vi "Write RS-xxx To GPIB ConvBox Data Structure.vi"(8 "error in (no error)":errorcluster, 10 "RS-xxx To GPIB ConvBox Data Structure":T1, 11 "Listener in":refnum<class "Listener.lvclass">) -> (0 "error out":errorcluster, 3 "Listener out":refnum<class "Listener.lvclass">)   [LabVIEW 2023, in "Listener.lvclass"]
uses:
  Listener.lvclass
  ListenerClassControls/RS-xxx To GPIB ConvBox Data Structure.ctl
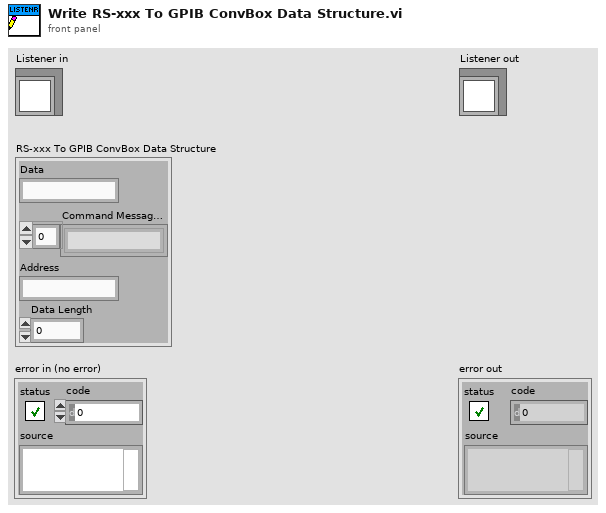
[diagram p1: front panel]
types:
  T1 = typedef "Listener.lvclass/RS-xxx To GPIB ConvBox Data Structure.ctl" = cluster{"Data":string, "Command Messages Read":string[], "Address":string, "Data Length":u32}
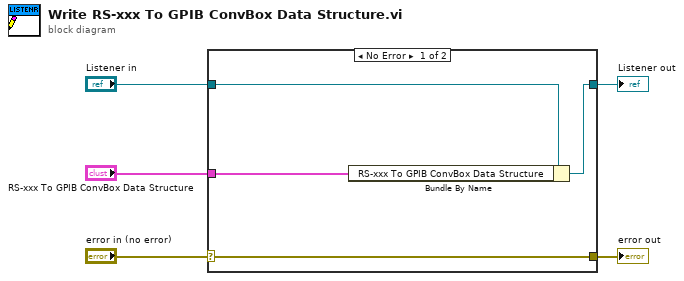
[diagram p0: block diagram]
diagram:
  n1 = case shown="No Error" "error in (no error)" {
    selector: "error in (no error)" -> [w9 w10]
    tunnel: [w9 w10] -> w4
    tunnel: [w7 w11] -> w2
    tunnel: "Listener in" -> [w8 w11]
    tunnel: "RS-xxx To GPIB ConvBox Data Structure" -> [w6 _]
    frame No Error {
      n2 = Bundle By Name(cluster=w8, "RS-xxx To GPIB ConvBox Data Structure"=w6) -> (w7:refnum<class "Listener.lvclass">)
    }
    frame Error {
    }
  }
  "error out" <- w4
  "Listener out" <- w2
